vi "ANC300_Filter.vi"(0 "ANC300 Communication Port In":refnum<visa-resource-name>="COM99", 1 "connection ID in":refnum<k5>, 2 "Axis":u8=1 min=1 max=6, 3 "filter input":dbl(ring)=16.0 items=["OFF"=0.0, "1,6 Hz"=1.6, "16 Hz"=16.0, "160 Hz"=160.0, "1600 Hz"=1600.0], 5 "error in":T1, 6 "set / get":bool=TRUE, 7 "Time to wait [ms]":u32=20) -> (12 "command string":string, 13 "data out":string, 14 "ANC300 Communication Port Out":refnum<visa-resource-name>="COM99", 15 "connection ID out":refnum<k5>, 16 "value out":string, 17 "filter":dbl(ring) items=["OFF"=0.0, "1,6 Hz"=1.6, "16 Hz"=16.0, "160 Hz"=160.0, "1600 Hz"=1600.0], 18 "transfer ok":bool=TRUE, 19 "error out":T1)   [LabVIEW 2022 SP3]
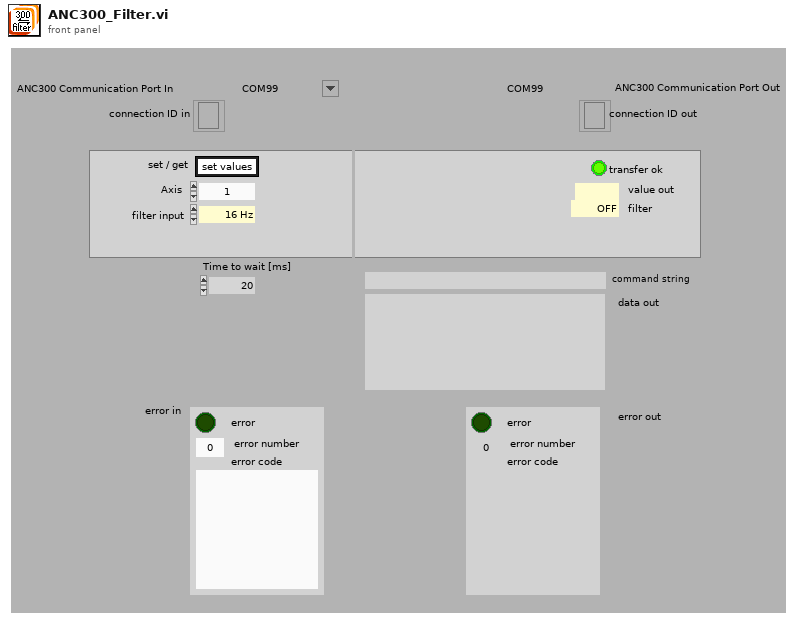
[diagram p1: front panel]
types:
  T1 = cluster{"error ":bool, "error number":i32, "error code":string}
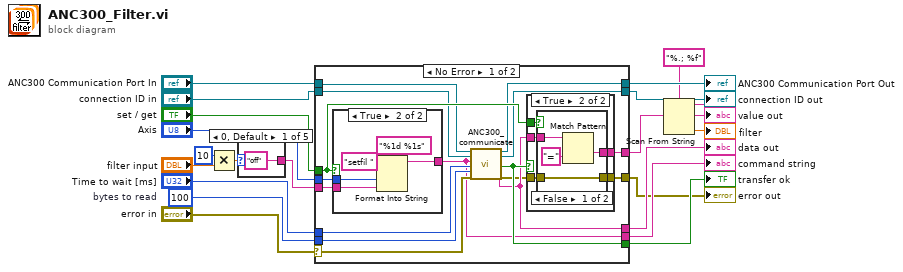
[diagram p0: block diagram]
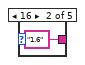
[diagram p2: hidden frame]
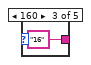
[diagram p3: hidden frame]
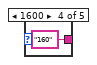
[diagram p4: hidden frame]
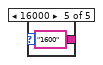
[diagram p5: hidden frame]
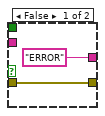
[diagram p6: hidden frame]
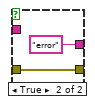
[diagram p7: hidden frame]
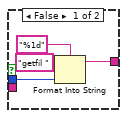
[diagram p8: hidden frame]
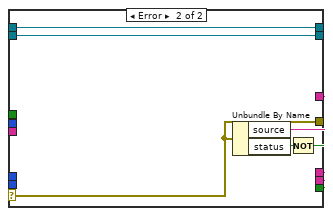
[diagram p9: hidden frame]
diagram:
  w15 = 100  # bytes to read
  n1 = Multiply(x=10, y="filter input") -> (x*y=w4:dbl)
  n2 = case shown="0, Default" w4 {
    tunnel: ["off" "1.6" "16" "160" "1600"] -> w1
    frame 0, Default {
    }
    frame 16 {
    }
    frame 160 {
    }
    frame 1600 {
    }
    frame 16000 {
    }
  }
  n3 = case shown="No Error" "error in" {
    selector: "error in" -> [w32 w65]
    tunnel: "Axis" -> [w41 _]
    tunnel: "set / get" -> [w40 _]
    tunnel: "ANC300 Communication Port In" -> [w39 w69]
    tunnel: "connection ID in" -> [w38 w68]
    tunnel: "Time to wait [ms]" -> [w37 _]
    tunnel: w15 -> [w36 _]
    tunnel: [w35 w64] -> w7
    tunnel: [w34 w69] -> w13
    tunnel: [w33 w68] -> w12
    tunnel: [w31 w66] -> w9
    tunnel: [w30 w64] -> w11
    tunnel: [w29 w64] -> w10
    tunnel: [w27 w65] -> w8
    tunnel: w1 -> [w26 _]
    frame No Error {
      n4 = case shown="True" w40 {
        tunnel: w41 -> [w55 w60]
        tunnel: [w56 w61] -> w30
        tunnel: w26 -> [_ w59]
        frame False {
          n5 = Format Into String(format string="%1d", initial string="getfil ", w55) -> (resulting string=w56:string)  [unwired: 1 in, 1 out]
        }
        frame True {
          n6 = Format Into String(format string="%1d %1s", initial string="setfil ", w60, w59) -> (resulting string=w61:string)  [unwired: 1 in, 1 out]
        }
      }
      n7 = call "ANC300_communicate.vi"("ANC300 Communication Port In"=w39, "connection ID in"=w38, "commando string"=w30, "Time to wait [ms]"=w37, "bytes to read"=w36, "error in"=w32) -> ("ANC300 Communication Port Out"=w34:refnum<visa-resource-name>, "connection ID out"=w33:refnum<k5>, "read data"=w29:string, "transfer ok"=w31:bool, "error out"=w28:T1)  [unwired: 9 in]
      n8 = case shown="True" w31 {
        tunnel: ["ERROR" w48] -> w35
        tunnel: w29 -> [_ w47]
        tunnel: w40 -> [_ w46]
        tunnel: w28 -> [w43 w45]
        tunnel: [w43 w44] -> w27
        frame False {
        }
        frame True {
          n9 = case shown="False" w46 {
            tunnel: w47 -> [w51 _]
            tunnel: [w50 "error" ("data out")] -> w48
            tunnel: w45 -> [w49 w54]
            tunnel: [w49 w54] -> w44
            frame False {
              n10 = Match Pattern(string=w51, regular expression="=") -> (after substring=w50:string)  [unwired: 1 in, 3 out]
            }
            frame True {
            }
          }
        }
      }
    }
    frame Error {
      n11 = Unbundle By Name(w65) -> ("source"=w64:string, "status"=w67:bool)
      n12 = Not(x=w67) -> (.not. x?=w66:bool)
    }
  }
  "data out" <- w10
  "connection ID out" <- w12
  "error out" <- w8
  "command string" <- w11
  "value out" <- w7
  "transfer ok" <- w9
  "ANC300 Communication Port Out" <- w13
  n13 = Scan From String(format string="%.; %f", input string=w7) -> (output 1=→"filter":dbl)  [unwired: 3 in, 3 out]
